vi "Begin.vi"(8 "error in":errorcluster, 10 "Image Size":T1=enum."320x240", 11 "RobotConfig":T2={"Motors"={"DriveLeftPrimary"={"CAN Address"=0, "Invert"=FALSE, "InvertSensor"=FALSE, "Unit Conversion Factor"=0.0, "Brake Mode"=enum."Override to Brake", "Reverse Limt Switch Mode"=enum."Normally Closed", "Forward Limt Swith Mode"=enum."Normally Closed"}, "DriveLeftSecondary1"={"CAN Address"=0, "Invert"=FALSE, "InvertSensor"=FALSE, "Unit Conversion Factor"=0.0, "Brake Mode"=enum."Override to Brake", "Reverse Limt Switch Mode"=enum."Normally Closed", "Forward Limt Swith Mode"=enum."Normally Closed"}, "DriveRightPrimary"={"CAN Address"=0, "Invert"=FALSE, "InvertSensor"=FALSE, "Unit Conversion Factor"=0.0, "Brake Mode"=enum."Override to Brake", "Reverse Limt Switch Mode"=enum."Normally Closed", "Forward Limt Swith Mode"=enum."Normally Closed"}, "DriveRightSecondary1"={"CAN Address"=0, "Invert"=FALSE, "InvertSensor"=FALSE, "Unit Conversion Factor"=0.0, "Brake Mode"=enum."Override to Brake", "Reverse Limt Switch Mode"=enum."Normally Closed", "Forward Limt Swith Mode"=enum."Normally Closed"}, "RightIntake"={"CAN Address"=0, "Invert"=FALSE, "InvertSensor"=FALSE, "Unit Conversion Factor"=0.0, "Brake Mode"=enum."Override to Brake", "Reverse Limt Switch Mode"=enum."Normally Closed", "Forward Limt Swith Mode"=enum."Normally Closed"}, "LeftIntake"={"CAN Address"=0, "Invert"=FALSE, "InvertSensor"=FALSE, "Unit Conversion Factor"=0.0, "Brake Mode"=enum."Override to Brake", "Reverse Limt Switch Mode"=enum."Normally Closed", "Forward Limt Swith Mode"=enum."Normally Closed"}, "ArmPivot"={"CAN Address"=0, "Invert"=FALSE, "InvertSensor"=FALSE, "Unit Conversion Factor"=0.0, "Brake Mode"=enum."Override to Brake", "Reverse Limt Switch Mode"=enum."Normally Closed", "Forward Limt Swith Mode"=enum."Normally Closed"}, "ArmExtend"={"CAN Address"=0, "Invert"=FALSE, "InvertSensor"=FALSE, "Unit Conversion Factor"=0.0, "Brake Mode"=enum."Override to Brake", "Reverse Limt Switch Mode"=enum."Normally Closed", "Forward Limt Swith Mode"=enum."Normally Closed"}, "ArmPivot2"={"CAN Address"=9, "Invert"=FALSE, "InvertSensor"=FALSE, "Unit Conversion Factor"=0.0, "Brake Mode"=enum."Override to Brake", "Reverse Limt Switch Mode"=enum."Normally Closed", "Forward Limt Swith Mode"=enum."Normally Closed"}, "Climber"={"CAN Address"=10, "Invert"=FALSE, "InvertSensor"=FALSE, "Unit Conversion Factor"=0.0, "Brake Mode"=enum."Override to Brake", "Reverse Limt Switch Mode"=enum."Disabled", "Forward Limt Swith Mode"=enum."Disabled"}}, "Sensors"={"IMU"={"Yaw Axis"=enum."Z", "SPI Bus"=enum."SPI MXP", "AHRS Algorithm"=enum."Complementary", "Calibration Time (s)"=3.0, "Calibrate On Open"=TRUE}, "LimitSwitch1"={"DIOChannel"=enum."DIO 0", "Active Low"=FALSE}, "LimitSwitch2"={"DIOChannel"=enum."DIO 0", "Active Low"=FALSE}, "BeamBreak"={"DIOChannel"=enum."DIO 0", "Active Low"=FALSE}, "JeVois"={"Baud Rate"=9600, "Parity"=0, "Data Bits"=8, "Stop Bits"=10, "Termination Char (0xA = '\\n' = LF)"=10, "Enable Termination Char? (T)"=TRUE, "Flow Control"=0, "Timeout Value (ms)"=5000, "Serial Port"=enum."Onboard RS-232"}}, "PID"={"ArmExtend"={"P"=0.0, "I"=0.0, "D"=0.0, "F"=0.0, "IZone"=0.0}, "ArmRotate"={"P"=0.0, "I"=0.0, "D"=0.0, "F"=0.0, "IZone"=0.0}, "Drive"={"P"=0.0, "I"=0.0, "D"=0.0, "F"=0.0, "IZone"=0.0}, "DriveGyro Kp ((in/sec)/deg)"=0.0}, "Solenoids"={"ArmClaw"={"Forward Channel"=enum."Solenoid 0", "Invert"=FALSE, "Reverse Channel"=enum."Solenoid 0"}, "IntakeExtend"={"Forward Channel"=enum."Solenoid 0", "Invert"=FALSE, "Reverse Channel"=enum."Solenoid 0"}, "IntakeOpen"={"Forward Channel"=enum."Solenoid 0", "Invert"=FALSE, "Reverse Channel"=enum."Solenoid 0"}, " Shifter"={"Forward Channel"=enum."Solenoid 0", "Invert"=FALSE, "Reverse Channel"=enum."Solenoid 0"}}, "RobotDimensions "={"Length"=0.0, "Height"=0.0, "HeightOfBumpers"=0.0, "DistanceFromFrameEdgeToPyramid "=0.0, "HeightOfFrameToIntake"=0.0, "EdgeOfFrameToOrigin"=0.0}, "ArmHomePosition"={"Angle (rad)"=0.0, "Radius (in)"=0.0}} {"Sensors"."JeVois"."Flow Control" items=["None", "XON/XOFF", "RTS/CTS", "XON/XOFF & RTS/CTS", "DTR/DSR", "XON/XOFF & DTR/DSR"]; "Sensors"."JeVois"."Termination Char (0xA = '\\n' = LF)" format="%.0x"; "Sensors"."JeVois"."Stop Bits" items=["1.0"=10, "1.5"=15, "2.0"=20]; "Sensors"."JeVois"."Parity" items=["None", "Odd", "Even", "Mark", "Space"]}) -> (0 "error out":errorcluster)   [LabVIEW 2017]
doc: "Called before other user functions, this VI is expected to open initial I/O refnums, load in file data, and do all program initialization. Notice that the <B>error out</B> terminal is simply used for data flow. Wiring it to other structures or subVIs ensures that this VI runs first."
uses:
  PowerUpSrc/TypeDefs/ConfigComponents/Config_Robot.ctl
  PowerUpSrc/TypeDefs/ConfigComponents/Config_Motor.ctl
  <vilib>/Rock Robotics/WPI/ThirdParty/Phoenix-LabVIEW/Motor Controller/Controls/CTRE_Phoenix_MotorControl_NeutralMode.ctl
  <vilib>/Rock Robotics/WPI/ThirdParty/Phoenix-LabVIEW/Motor Controller/Controls/CTRE_Phoenix_MotorControl_LimitSwitchNormal.ctl
  PowerUpSrc/TypeDefs/ConfigComponents/Config_IMU.ctl
  <vilib>/Rock Robotics/SystemInterfaces/spilib/spi_bus.ctl
  PowerUpSrc/TypeDefs/ConfigComponents/Config_DigitalIO.ctl
  <vilib>/Rock Robotics/SystemInterfaces/DIO/FPGA_DIOChannel.ctl
  PowerUpSrc/TypeDefs/ConfigComponents/Config_SerialPort.ctl
  <vilib>/Rock Robotics/WPI/SerialPort/WPI_SerialPort.ctl
  PowerUpSrc/TypeDefs/ConfigComponents/Config_PIDParams.ctl
  PowerUpSrc/TypeDefs/ConfigComponents/Config_DoubleSolenoid.ctl
  <vilib>/Rock Robotics/WPI/Solenoid/WPI_SolenoidChannel.ctl
  PowerUpSrc/TypeDefs/ConfigComponents/Config_Dimensions.ctl
  PowerUpSrc/TypeDefs/ConfigComponents/Config_ArmHome.ctl
  <vilib>/Rock Robotics/WPI/Camera/WPI_CameraImageSize.ctl
  <vilib>/Rock Robotics/WPI/DriverStation/WPI_DriverStationRobotMode2.ctl
  <vilib>/Rock Robotics/SystemInterfaces/i2clib/i2c_bus.ctl
  Robot Global Data.vi
  <vilib>/Rock Robotics/Network Tables/NT Write String Array.vi
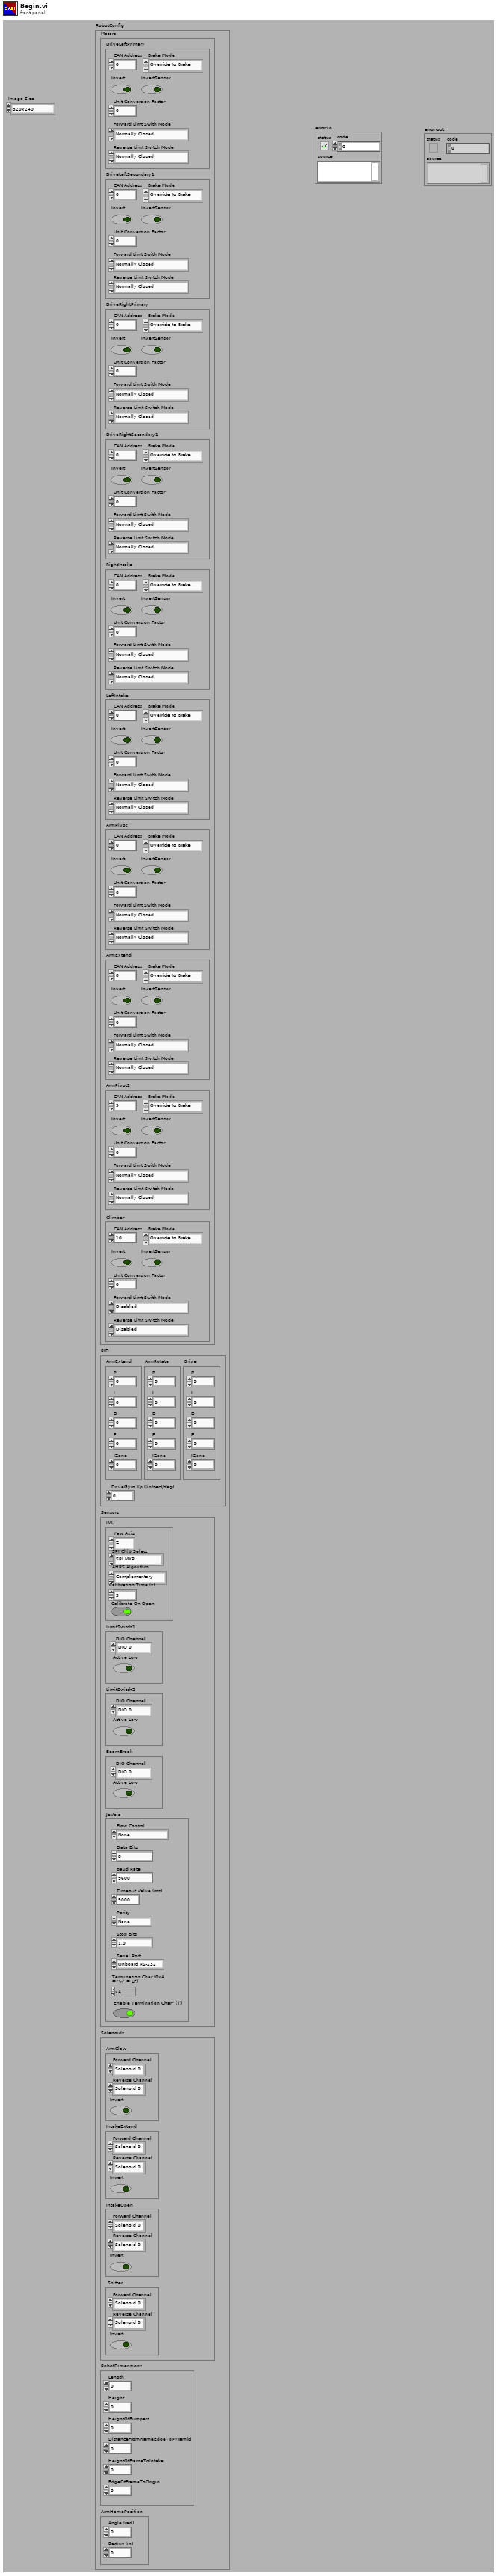
[diagram p1: front panel]
types:
  T1 = typedef "WPI_CameraImageSize.ctl" = enum16{"640x480", "320x240", "160x120", "Custom"}
  T2 = typedef "Config_Robot.ctl" = cluster{"Motors":cluster{"DriveLeftPrimary":T3, "DriveLeftSecondary1":T3, "DriveRightPrimary":T3, "DriveRightSecondary1":T3, "RightIntake":T3, "LeftIntake":T3, "ArmPivot":T3, "ArmExtend":T3, "ArmPivot2":T3, "Climber":T3}, "Sensors":cluster{"IMU":T6, "LimitSwitch1":T8, "LimitSwitch2":T8, "BeamBreak":T8, "JeVois":T10}, "PID":cluster{"ArmExtend":T12, "ArmRotate":T12, "Drive":T12, "DriveGyro Kp ((in/sec)/deg)":dbl}, "Solenoids":cluster{"ArmClaw":T13, "IntakeExtend":T13, "IntakeOpen":T13, " Shifter":T13}, "RobotDimensions ":T15, "ArmHomePosition":T16}
  T3 = typedef "Config_Motor.ctl" = cluster{"CAN Address":u8, "Invert":bool, "InvertSensor":bool, "Unit Conversion Factor":dbl, "Brake Mode":T4, "Reverse Limt Switch Mode":T5, "Forward Limt Swith Mode":T5}
  T4 = typedef "CTRE_Phoenix_MotorControl_NeutralMode.ctl" = enum8{"EEPROMSetting", "Override to Coast", "Override to Brake"}
  T5 = typedef "CTRE_Phoenix_MotorControl_LimitSwitchNormal.ctl" = enum16{"Normally Open", "Normally Closed", "Disabled"}
  T6 = typedef "Config_IMU.ctl" = cluster{"Yaw Axis":enum16{"X", "Y", "Z"}, "SPI Bus":T7, "AHRS Algorithm":enum16{"Complementary", "Madgwick"}, "Calibration Time (s)":dbl, "Calibrate On Open":bool}
  T7 = typedef "spi_bus.ctl" = enum16{"SPI On-Board, CS0", "SPI On-Board, CS1", "SPI On-Board, CS2", "SPI On-Board, CS3", "SPI MXP", "Invalid"}
  T8 = typedef "Config_DigitalIO.ctl" = cluster{"DIOChannel":T9, "Active Low":bool}
  T9 = typedef "FPGA_DIOChannel.ctl" = enum8{"DIO 0", "DIO 1", "DIO 2", "DIO 3", "DIO 4", "DIO 5", "DIO 6", "DIO 7", "DIO 8", "DIO 9", "DIO MXP 0", "DIO MXP 1", "DIO MXP 2", "DIO MXP 3", "DIO MXP 4", "DIO MXP 5", "DIO MXP 6", "DIO MXP 7", "DIO MXP 8", "DIO MXP 9", "DIO MXP 10", "DIO MXP 11", "DIO MXP 12", "DIO MXP 13", "DIO MXP 14", "DIO MXP 15", "SPI Port CS1", "SPI Port CS2", "SPI Port CS3", "SPI Port MISO", "SPI Port MOSI", "Invalid"}
  T10 = typedef "Config_SerialPort.ctl" = cluster{"Baud Rate":u32, "Parity":u16, "Data Bits":u16, "Stop Bits":u16, "Termination Char (0xA = '\\n' = LF)":u8, "Enable Termination Char? (T)":bool, "Flow Control":u16, "Timeout Value (ms)":u32, "Serial Port":T11}
  T11 = typedef "WPI_SerialPort.ctl" = enum16{"Onboard RS-232", "MXP TTL", "USB 1", "USB 2"}
  T12 = typedef "Config_PIDParams.ctl" = cluster{"P":dbl, "I":dbl, "D":dbl, "F":dbl, "IZone":dbl}
  T13 = typedef "Config_DoubleSolenoid.ctl" = cluster{"Forward Channel":T14, "Invert":bool, "Reverse Channel":T14}
  T14 = typedef "WPI_SolenoidChannel.ctl" = enum8{"Solenoid 0", "Solenoid 1", "Solenoid 2", "Solenoid 3", "Solenoid 4", "Solenoid 5", "Solenoid 6", "Solenoid 7", "Invalid"}
  T15 = typedef "Config_Dimensions.ctl" = cluster{"Length":dbl, "Height":dbl, "HeightOfBumpers":dbl, "DistanceFromFrameEdgeToPyramid ":dbl, "HeightOfFrameToIntake":dbl, "EdgeOfFrameToOrigin":dbl}
  T16 = typedef "Config_ArmHome.ctl" = cluster{"Angle (rad)":dbl, "Radius (in)":dbl}
  T17 = typedef "i2c_bus.ctl" = enum16{"I2C On-Board", "I2C MXP", "Invalid"}
  T18 = typedef "WPI_DriverStationRobotMode2.ctl" = enum16{"Autonomous Disabled", "Autonomous Enabled", "Teleop Disabled", "Teleop Enabled", "Disconnected", "Finish", "Test Disabled", "Test Enabled", "Emergency Stopped"}
  T19 = typedef "WPI_I2CDevRef.ctl" = cluster{"DevStatus":errorcluster, "Device Address":u8, "Handle":i32, "I2C Bus":T17}
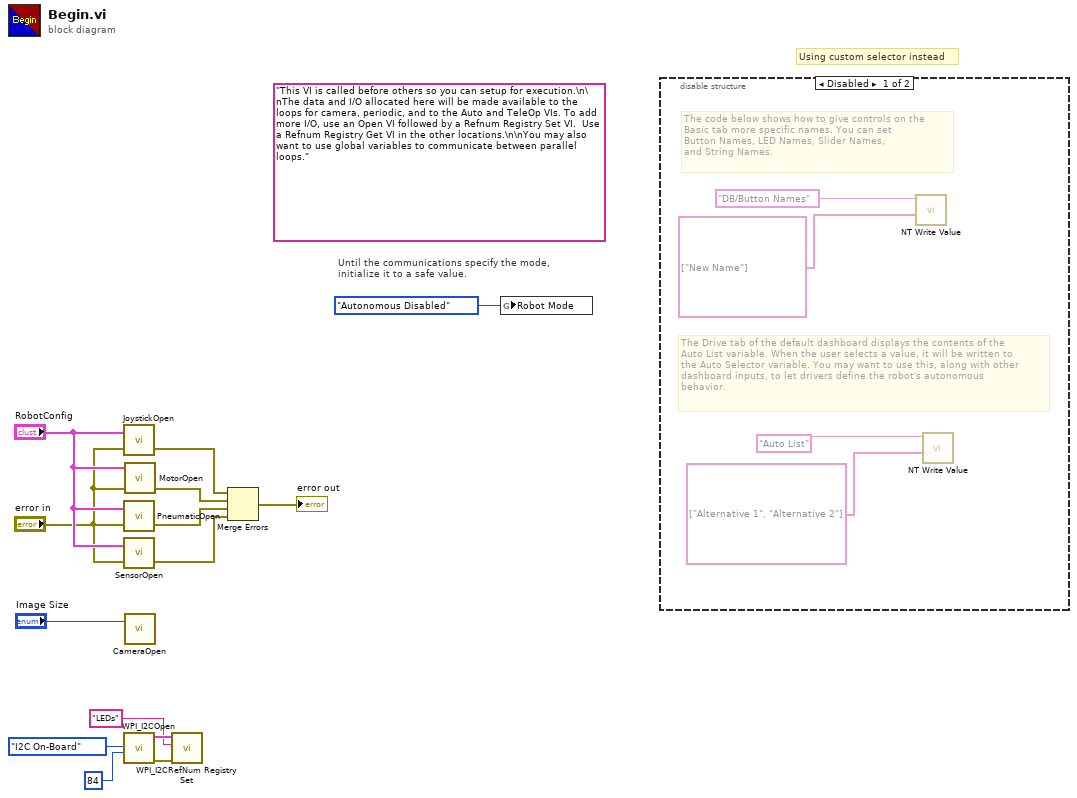
[diagram p0: block diagram]
diagram:
  (unwired) "This VI is called before others so you can setup for execution.\n\nThe data and I/O allocated here will be made available to the loops for camera, periodic, and to the Auto and TeleOp VIs. To add more I/O, use an Open VI followed by a Refnum Registry Set VI.  Use a Refnum Registry Get VI in the other locations.\n\nYou may also want to use global variables to communicate between parallel loops."
  # "Using custom selector instead"
  # "Until the communications specify the mode,\ninitialize it to a safe value."
  n1 = call "JoystickOpen.vi"("error in"="error in", "RobotConfig"="RobotConfig") -> ("error out"=w11:errorcluster)  [unwired: 1 in]
  n2 = call "PneumaticOpen.vi"("error in (no error)"="error in", "RobotConfig"="RobotConfig") -> ("error out"=w12:errorcluster)  [unwired: 1 in]
  n3 = call "SensorOpen.vi"("error in (no error)"="error in", "RobotConfig"="RobotConfig") -> ("error out"=w13:errorcluster)  [unwired: 1 in]
  n4 = call <vilib>:"WPI_I2COpen.vi"("Device Address"=u8 84, "I2C Bus"=i2c_bus."I2C On-Board") -> ("error out"=w5:errorcluster, "I2CDevRef"=w4:T19)  [unwired: 8 in]
  n5 = call "MotorOpen.vi"("error in (no error)"="error in", "RobotConfig"="RobotConfig") -> ("error out"=w9:errorcluster)  [unwired: 1 in, 2 out]
  n6 = call "CameraOpen.vi"("Image Size"="Image Size") -> ()  [unwired: 2 in, 1 out]
  n7 = call <vilib>:"WPI_I2CRefNum Registry Set.vi"("error in (no error)"=w5, "refnum name"="LEDs", "I2CDevRef"=w4) -> ()  [unwired: 7 in, 2 out]
  n8 = Merge Errors(w11, w9, w12, w13) -> (→"error out":errorcluster)
  n9 = global write "Robot Global Data.vi" "Robot Mode"(WPI_DriverStationRobotMode2."Autonomous Disabled" ("Robot Mode")) -> ()
  n10 = disable-structure shown="Disabled" {
    frame Disabled {
      # "The Drive tab of the default dashboard displays the contents of the\nAuto List variable. When the user selects a value, it will be written to\nthe Auto Selector variable. You may want to use this, along with other\ndashboard inputs, to let drivers define the robot's autonomous\nbehavior."
      # "The code below shows how to give controls on the\nBasic tab more specific names. You can set\nButton Names, LED Names, Slider Names,\nand String Names."
      n11 = call-poly <vilib>:"NT Write Value.vi"("String Array"=string[] ["New Name"], "Name"="DB/Button Names") -> ()  [unwired: 9 in, 1 out]
      n12 = call-poly <vilib>:"NT Write Value.vi"("String Array"=string[] ["Alternative 1", "Alternative 2"], "Name"="Auto List") -> ()  [unwired: 9 in, 1 out]
    }
    frame Enabled {
    }
  }
